vi "PLC_comm.vi"() -> ()   [LabVIEW 2018]
uses:
  <vilib>/OPCUA/controls/NodeId.ctl
  <vilib>/OPCUA/NI OPC UA Client.lvlib
panel:
  in  "Value":bool
  out "PLC error out":errorcluster
  in  "Direction":bool
  in  "Relative Motor position PLC":dbl
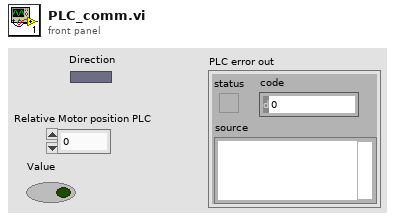
[diagram p1: front panel]
types:
  T1 = cluster{"message mode":enum16{"None", "Sign", "Sign and Encrypt"}, "security":enum16{"Basic256", "Basic128Rsa15"}}
  T2 = typedef "NodeId.ctl" = string
  T3 = typedef "OPC UA Client Refnum.ctl" = refnum<k21>
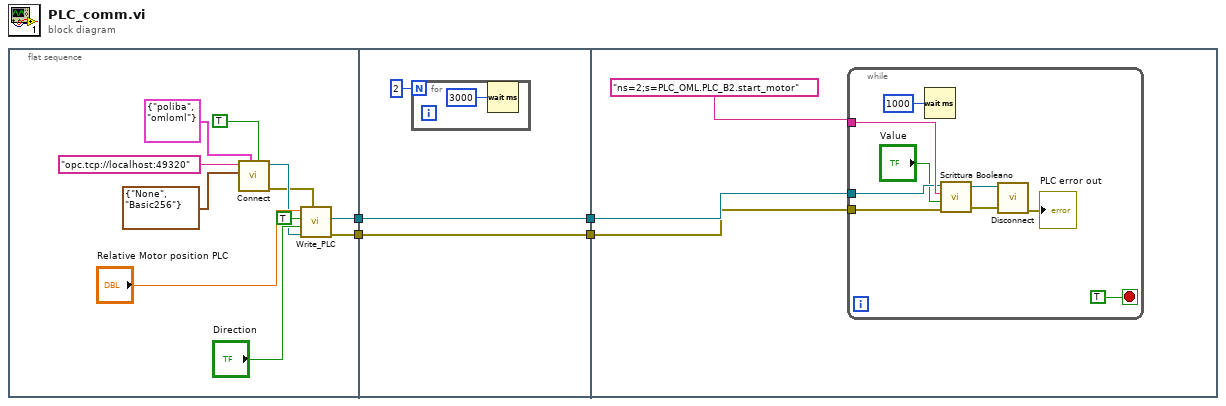
[diagram p0: block diagram]
diagram:
  n1 = flat-sequence {
    tunnel: [w7] -> w4
    tunnel: [w6] -> w2
    tunnel: w4 -> [w18]
    tunnel: [w18] -> w3
    tunnel: w2 -> [w17]
    tunnel: [w17] -> w1
    tunnel: w3 -> [w22]
    tunnel: w1 -> [w21]
    frame #0 {
      n2 = call <vilib>:"Connect.vi"("trust any server (F)"=TRUE, "username/password"=cluster{"username":string, "password":string} {"username"="poliba", "password"="omloml"}, "security policy"=T1 {"message mode"=enum."None", "security"=enum."Basic256"}, "server endpoint URL"="opc.tcp://localhost:49320") -> ("error out"=w8:errorcluster, "OPC UA client refnum out"=w9:T3)  [unwired: 5 in, 1 out]
      n3 = call "Write_PLC.vi"("error in"=w8, "OPC UA client refnum out"=w9, "Direction"="Direction", "Start_communication"=TRUE, "Relative_Motor_position"="Relative Motor position PLC") -> ("error out"=w6:errorcluster, "OPC UA client refnum out 2"=w7:T3)  [unwired: 2 out]
    }
    frame #1 {
      n4 = for {
        N: 2 -> [_]
        n5 = Wait (ms)(milliseconds to wait=u32 3000) -> ()  [unwired: 1 out]
      }
    }
    frame #2 {
      n6 = while {
        tunnel: T2 "ns=2;s=PLC_OML.PLC_B2.start_motor" ("node ID") -> [w28]
        tunnel: w22 -> [w27]
        tunnel: w21 -> [w26]
        stop <- TRUE stop-if-true
        n7 = Wait (ms)(milliseconds to wait=u32 1000) -> ()  [unwired: 1 out]
        n8 = call "Scrittura Booleano.vi"("OPC UA client refnum in"=w27, "node ID"=w28, "Value"="Value", "error in (no error)"=w26) -> ("OPC UA client refnum out"=w30:T3, "error out"=w29:errorcluster)  [unwired: 1 in, 1 out]
        n9 = call <vilib>:"Disconnect.vi"("error in (no error)"=w29, "OPC UA client refnum in"=w30) -> ("error out"=→"PLC error out":errorcluster)  [unwired: 9 in]
      }
    }
  }
